vi "Send to CS.vi"(8 "error in (no error)":errorcluster, 10 "String to write":string, 11 "TCS in":refnum<class "TCS.lvclass">) -> (0 "error out":errorcluster, 3 "TCS out":refnum<class "TCS.lvclass">)   [LabVIEW 2013, in "TCS.lvclass"]
uses:
  Lib.llb/TCS.lvclass
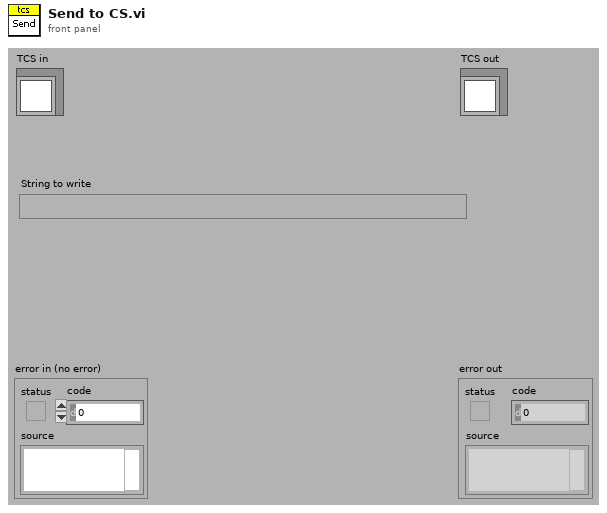
[diagram p1: front panel]
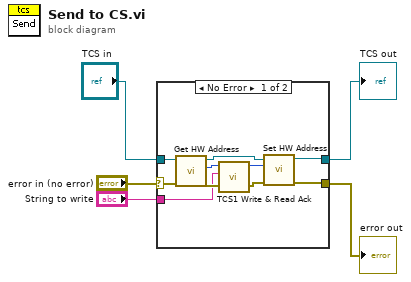
[diagram p0: block diagram]
diagram:
  n1 = case shown="No Error" "error in (no error)" {
    selector: "error in (no error)" -> [w13 w17]
    tunnel: [w10 w17] -> w5
    tunnel: [w8 w16] -> w4
    tunnel: "String to write" -> [w6 _]
    tunnel: "TCS in" -> [w15 w16]
    frame No Error {
      n2 = call-dynamic "Get HW Address.vi"("error in (no error)"=w13, "CS.lvclass in"=w15) -> ("error out"=w12:errorcluster, "HW Address"=w14:i32, "CS.lvclass out"=w9:refnum<class "TCS.lvclass">)  [unwired: 7 in]
      n3 = call "TCS1 Write & Read Ack.vi"("port number (1:com2)"=w14, "write buffer"=w6, "error in"=w12) -> ("port number out"=w7:u16, "error out"=w11:errorcluster)  [unwired: 2 in, 1 out]
      n4 = call-dynamic "Set HW Address.vi"("error in (no error)"=w11, "HW Address"=w7, "CS.lvclass in"=w9) -> ("error out"=w10:errorcluster, "CS.lvclass out"=w8:refnum<class "TCS.lvclass">)  [unwired: 7 in]
    }
    frame Error {
    }
  }
  "error out" <- w5
  "TCS out" <- w4
